vi "Register API.vi"(8 "error in (no error)":errorcluster, 10 "API":refnum<class "API.lvclass">, 11 "VolatusCore in":refnum<class "VolatusCore.lvclass">) -> (0 "error out":errorcluster, 3 "VolatusCore out":refnum<class "VolatusCore.lvclass">)   [LabVIEW 2020, in "Volatus.lvlib" / "VolatusCore.lvclass"]
uses:
  VolatusCore.lvclass
  VolatusCore.lvclass/VolatusCore.ctl
  Identity/Identity.lvclass
  API/API.lvclass
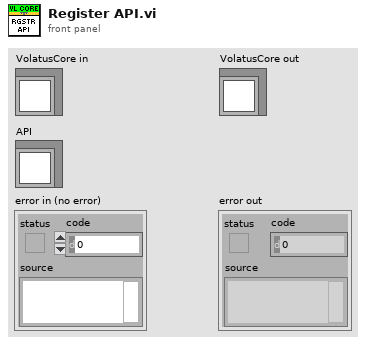
[diagram p1: front panel]
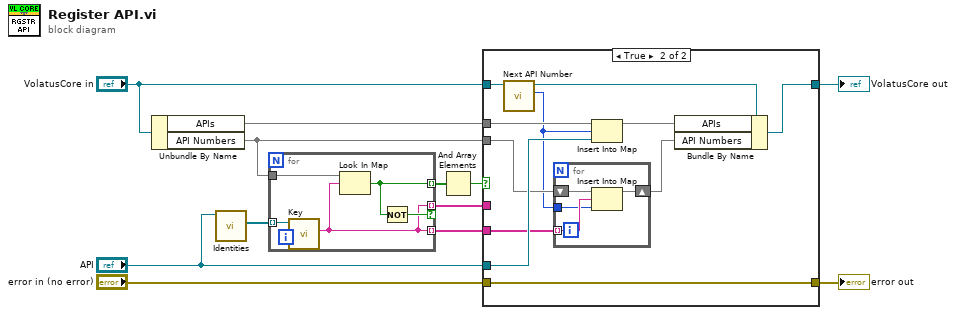
[diagram p0: block diagram]
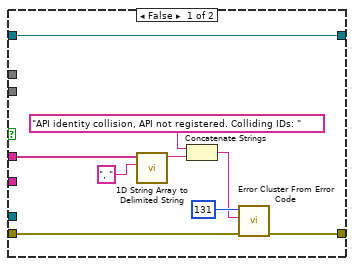
[diagram p2: hidden frame]
diagram:
  n1 = Unbundle By Name("VolatusCore in") -> ("APIs"=w3:map{u32, refnum<class "API.lvclass">}, "API Numbers"=w9:map{string, u32})
  n2 = call-dynamic "Identities.vi"("API in"="API") -> ("Identities"=w12:refnum<class "Identity.lvclass">[])  [unwired: 8 in, 2 out]
  n3 = for {
    tunnel: w12 -> [w16] mode=indexing
    tunnel: w9 -> [w17]
    tunnel: [w15] -> w11 mode=indexing
    tunnel: [w13] -> w6 mode=indexing if=w14
    tunnel: [w13] -> w4 mode=indexing
    n4 = call "Key.vi"("Identity in"=w16) -> ("Key"=w13:string)  [unwired: 10 in]
    n5 = Look In Map(map=w17, key=w13) -> (key not found?=w15:bool)  [unwired: 1 in, 1 out]
    n6 = Not(x=w15) -> (.not. x?=w14:bool)
  }
  n7 = And Array Elements(Boolean array=w11) -> (logical AND=w10:bool)
  n8 = case shown="True" w10 {
    tunnel: w9 -> [_ w33]
    tunnel: "VolatusCore in" -> [w18 w37]
    tunnel: "error in (no error)" -> [w26 w27]
    tunnel: w6 -> [w25 _]
    tunnel: [w19 w27] -> w5
    tunnel: w4 -> [_ w34]
    tunnel: w3 -> [_ w36]
    tunnel: "API" -> [_ w35]
    tunnel: [w18 w28] -> w1
    frame False {
      n9 = call <vilib>:"1D String Array to Delimited String.vi"("delimiter"=", ", "string array"=w25) -> ("delimited string"=w22:string)  [unwired: 9 in]
      n10 = Concatenate Strings("API identity collision, API not registered. Colliding IDs: ", w22) -> (w20:string)
      n11 = call <vilib>:"Error Cluster From Error Code.vi"("error in (no error)"=w26, "error message (\"\")"=w20, "error code (0)"=131) -> ("error out"=w19:errorcluster)  [unwired: 6 in]
    }
    frame True {
      n12 = call "Next API Number.vi"("VolatusCore in"=w37) -> ("Next API"=w32:u32, "VolatusCore out"=w31:refnum<class "VolatusCore.lvclass">)  [unwired: 9 in]
      n13 = for {
        tunnel: w34 -> [w39] mode=indexing
        shift-right: [w40] -> w29
        shift-left: w33 -> [w41]
        tunnel: w32 -> [w38]
        n14 = Insert Into Map(map in=w41, key=w39, value=w38) -> (map out=w40:map{string, u32})  [unwired: 2 out]
      }
      n15 = Insert Into Map(map in=w36, key=w32, value=w35) -> (map out=w30:map{u32, refnum<class "API.lvclass">})  [unwired: 2 out]
      n16 = Bundle By Name(cluster=w31, "APIs"=w30, "API Numbers"=w29) -> (w28:refnum<class "VolatusCore.lvclass">)
    }
  }
  "error out" <- w5
  "VolatusCore out" <- w1
